vi "Is Invalid Waveform Element.vi"(8 "error in (no error)":errorcluster, 10 "element value (0.0)":dbl format="%.4f", 11 "CS++Scope":refnum<class "CS++Scope.lvclass">) -> (0 "error out":errorcluster, 2 "is invalid":bool, 3 "CS++Scope out":refnum<class "CS++Scope.lvclass">)   [LabVIEW 2016, in "CS++Scope.lvlib" / "CS++Scope.lvclass"]
doc: "After the read and fetch waveform VIs execute, each element in the waveform array contains either a voltage or a value indicating that the oscilloscope could not sample a voltage. The driver uses an IEEE defined NaN (Not a Number) value to mark as invalid each element in the waveform array for which the oscilloscope could not sample a voltage. This VI determines whether a value you pass from the waveform array is invalid."
uses:
  CS++Scope.lvclass
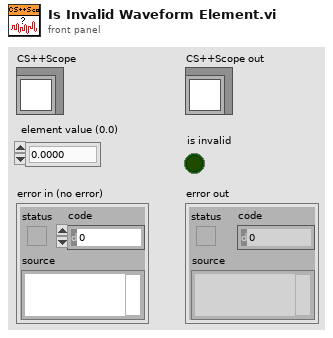
[diagram p1: front panel]
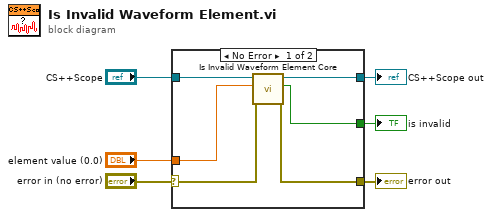
[diagram p0: block diagram]
diagram:
  n1 = case shown="No Error" "error in (no error)" {
    selector: "error in (no error)" -> [w11 w14]
    tunnel: [w10 w14] -> w5
    tunnel: [w8 w13] -> w3
    tunnel: "CS++Scope" -> [w9 w13]
    tunnel: "element value (0.0)" -> [w12 _]
    tunnel: [w7 _] -> w1
    frame No Error {
      n2 = call-dynamic "Is Invalid Waveform Element Core.vi"("error in (no error)"=w11, "element value (0.0)"=w12, "CS++Scope"=w9) -> ("error out"=w10:errorcluster, "is invalid"=w7:bool, "CS++Scope out"=w8:refnum<class "CS++Scope.lvclass">)  [unwired: 6 in]
    }
    frame Error {
    }
  }
  "error out" <- w5
  "is invalid" <- w1
  "CS++Scope out" <- w3
